vi "EnableOutput.vi"(8 "error in (no error)":errorcluster, 10 "gRPCid":T4, 11 "ctet_smu":T1) -> (0 "error out":errorcluster, 3 "ctet_smu out":T1)   [LabVIEW 2019, in "ctet_smu User Library.lvlib"]
uses:
  ctet_smu User Library.lvlib
  Servers/ctet_smu/gRPC lvSupport/Server API/typeDefs/grpcId.ctl
  Types/ctet_smu.ctl
  Servers/ctet_smu/ctet_smu Class/RPC Messages/measurementservice_SMUConfigResponse/measurementservice_SMUConfigResponse_Data.ctl
  Servers/ctet_smu/ctet_smu Class/RPC Messages/measurementservice_ErrorOut/measurementservice_ErrorOut_Data.ctl
  Servers/ctet_smu/ctet_smu Class/RPC Messages/measurementservice_SMUEnableResponse/measurementservice_SMUEnableResponse_Data.ctl
  Servers/ctet_smu/ctet_smu Class/ctet_smu.lvclass
  Servers/ctet_smu/gRPC lvSupport/gprc-lvsupport.lvlib
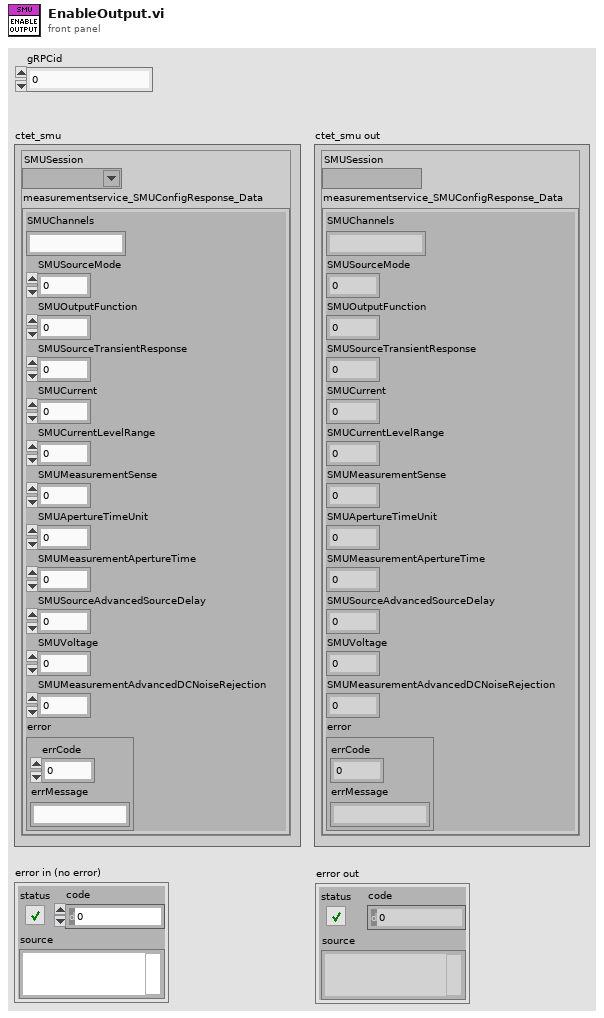
[diagram p1: front panel]
types:
  T1 = typedef "ctet_smu User Library.lvlib/ctet_smu.ctl" = cluster{"SMUSession":refnum<k15>, "measurementservice_SMUConfigResponse_Data":T2}
  T2 = typedef "ctet_smu.lvlib/ctet_smu.lvclass/measurementservice_SMUConfigResponse_Data.ctl" = cluster{"SMUChannels":string, "SMUSourceMode":i64, "SMUOutputFunction":i64, "SMUSourceTransientResponse":i64, "SMUCurrent":dbl, "SMUCurrentLevelRange":dbl, "SMUMeasurementSense":i64, "SMUApertureTimeUnit":i64, "SMUMeasurementApertureTime":dbl, "SMUSourceAdvancedSourceDelay":dbl, "SMUVoltage":dbl, "SMUMeasurementAdvancedDCNoiseRejection":i64, "error":T3}
  T3 = typedef "ctet_smu.lvlib/ctet_smu.lvclass/measurementservice_ErrorOut_Data.ctl" = cluster{"errCode":i64, "errMessage":string}
  T4 = typedef "ctet_smu.lvlib/gprc-lvsupport.lvlib/grpcId.ctl" = u64
  T5 = typedef "ctet_smu.lvlib/ctet_smu.lvclass/measurementservice_SMUEnableResponse_Data.ctl" = cluster{"error":T3}
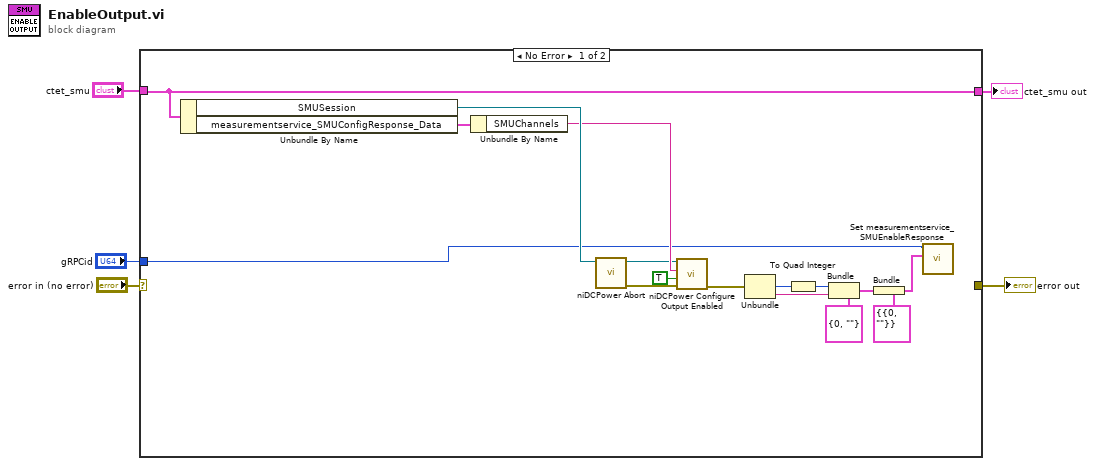
[diagram p0: block diagram]
diagram:
  n1 = case shown="No Error" "error in (no error)" {
    selector: "error in (no error)" -> [_ w23]
    tunnel: [_ w23] -> w5
    tunnel: "gRPCid" -> [w10 _]
    tunnel: "ctet_smu" -> [w20 w22]
    tunnel: [w20 w22] -> w1
    frame No Error {
      n2 = Unbundle By Name(w20) -> ("SMUSession"=w21:refnum<k15>, "measurementservice_SMUConfigResponse_Data"=w16:T2)
      n3 = Unbundle By Name(w16) -> ("SMUChannels"=w13:string)
      n4 = call <instrlib>:"niDCPower Abort.vi"("instrument handle"=w21) -> ("error out"=w15:errorcluster, "instrument handle out"=w12:refnum<k15>)  [unwired: 9 in]
      n5 = call <instrlib>:"niDCPower Configure Output Enabled.vi"("error in (no error)"=w15, "output enabled"=TRUE, "channel name"=w13, "instrument handle"=w12) -> ("error out"=w11:errorcluster)  [unwired: 6 in, 1 out]
      n6 = Unbundle(w11) -> ("code"=w18:i32, "source"=w19:string)  [unwired: 1 out]
      n7 = To Quad Integer(1:w18) -> (0:w17:i64)
      n8 = Bundle(cluster=T3 {"errCode"=0, "errMessage"=""} ("error"), "errCode"=w17, "errMessage"=w19) -> (w6:T3)
      n9 = Bundle(cluster=T5 {"error"={"errCode"=0, "errMessage"=""}} ("measurementservice_SMUEnableResponse_Data"), "error"=w6) -> (w8:T5)
      n10 = call "Set measurementservice_SMUEnableResponse.vi"("Message Data"=w8, "gRPCid"=w10) -> ()  [unwired: 9 in, 1 out]
    }
    frame Error {
    }
  }
  "error out" <- w5
  "ctet_smu out" <- w1
